vi "Python_node.vi"() -> ()   [LabVIEW 2018]
uses:
  <vilib>/Utility/file.llb/Read Delimited Spreadsheet (DBL).vi
panel:
  out "return value":dbl[][](array[numeric])
  in  "Array":dbl[][](array[numeric])
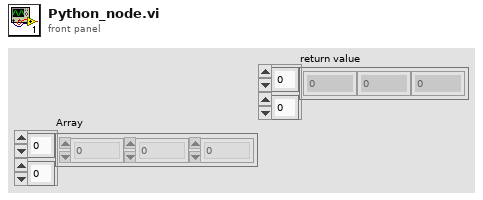
[diagram p1: front panel]
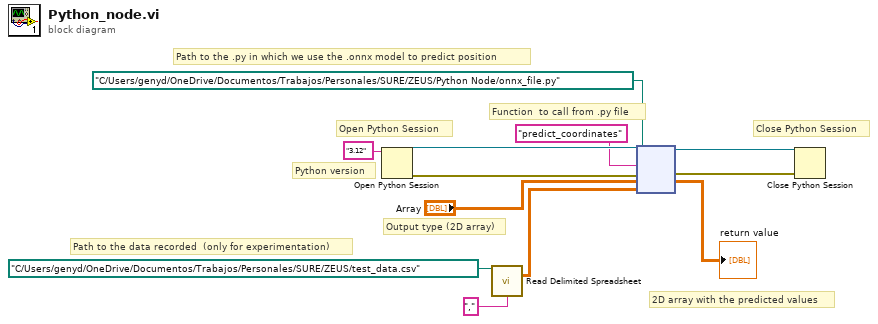
[diagram p0: block diagram]
diagram:
  # "Function  to call from .py file"
  # "2D array with the predicted values"
  # "Output type (2D array)"
  # "Close Python Session"
  # "Path to the data recorded  (only for experimentation)"
  # "Open Python Session"
  # "Python version"
  # "Path to the .py in which we use the .onnx model to predict position"
  n1 = Open Python Session(python version="3.12" ("Python version")) -> (session out=w10:refnum<k35>, error out=w9:errorcluster)  [unwired: 2 in]
  n2 = call-poly <vilib>:"Read Delimited Spreadsheet.vi"("file path (dialog if empty)"=path "C:/Users/genyd/OneDrive/Documentos/Trabajos/Personales/SURE/ZEUS/test_data.csv", "delimiter (\\t)"="," ("delimiter (\\t)")) -> ("all rows"=w4:dbl[][])  [unwired: 8 in, 5 out]
  n3 = node(w10, path "C:/Users/genyd/OneDrive/Documentos/Trabajos/Personales/SURE/ZEUS/Python Node/onnx_file.py" ("module path"), "predict_coordinates" ("function name"), w9, "Array", w4) -> (w12:refnum<k35>, w11:errorcluster, →"return value":dbl[][])  [unwired: 1 in, 2 out]
  n4 = Close Python Session(session in=w12, error in=w11) -> ()  [unwired: 1 out]
